vi "step loop.vi"(8 "error in (no error)":errorcluster, 11 "TapeDrive in":refnum<class "TapeDrive.lvclass">) -> (0 "error out":errorcluster, 1 "Boolean":bool, 2 "trajectories":dbl[][](graph)=[[1.0, 0.7046880791959296, 0.4965852858533471, 0.3499377259476329, 0.2465969370957652, 0.1737739140097176, 0.12245639698366893, 0.08629355394147512, 0.06081002915927391, 0.0628100291592739, 0.0648100291592739, 0.0668100291592739, 0.06881002915927391, 0.08881002915927391, 0.12881002915927392, 0.18881002915927392, 0.26881002915927393, 0.36881002915927397, 0.48881002915927396, 0.628810029159274, 0.788810029159274, 0.968810029159274, 1.0], [0.0, 0.0, 0.0, 0.0, 0.0, 0.0, 0.004000000000814907, 0.002999999998792191, 0.040000000000873115, 0.20499999999992724, 0.363999999999578, 0.5879999999997381, 0.7160000000003492, 0.7360000000007858, 0.7879999999986467, 0.6760000000012951, 0.3989999999994325, 0.01300000000082946, 0.004000000000814907, 0.003999999998995918, 0.0, 0.0, 0.0], [0.0, 0.0, 0.0, 0.0, 0.0, 0.0, 0.004000000000814907, -0.0010000000020227162, 0.037000000002080924, 0.16499999999905413, 0.15899999999965075, 0.22400000000016007, 0.12800000000061118, 0.020000000000436557, 0.05199999999786087, -0.11199999999735155, -0.27700000000186265, -0.385999999998603, -0.009000000000014552, -1.8189894035458565e-12, -0.003999999998995918, 0.0, 0.0]], 3 "TapeDrive out":refnum<class "TapeDrive.lvclass">, 4 "Slave":i32, 5 "VISA Refnum out":refnum<visa-resource-name>)   [LabVIEW 2020, in "TapeDrive.lvclass"]
uses:
  TapeDrive.lvclass
  TapeDrive.lvclass/TapeDrive.ctl
  shared/CompressAndUpdate(Poly)/CompressAndUpdate(Numeric).vi
  Newport ESP301/Newport ESP301.lvlib
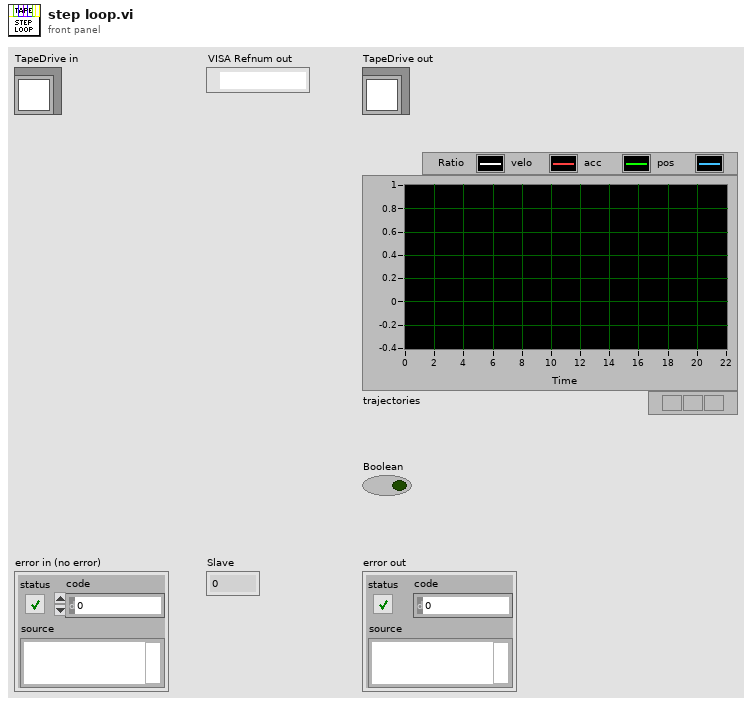
[diagram p1: front panel]
types:
  T1 = typedef "Direction_TypDef.ctl" = enum16{"left", "right"}
  T2 = cluster{"increase":dbl, "min velocity":dbl, "max velocity":dbl, "Stop increase":dbl}
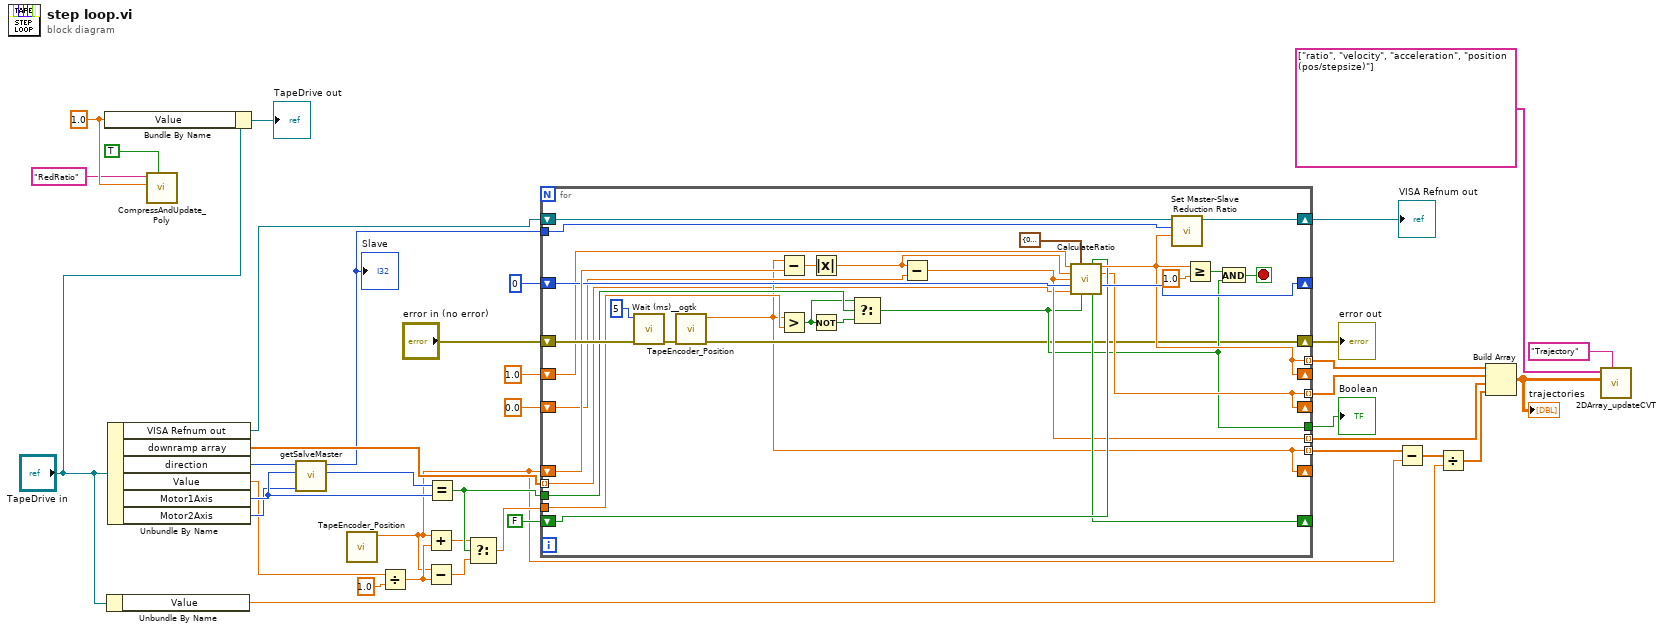
[diagram p0: block diagram]
diagram:
  w33 = 1.0 ("Reduction Ratio (0)")
  n1 = Bundle By Name(cluster="TapeDrive in", "Value"=w33) -> (→"TapeDrive out":refnum<class "TapeDrive.lvclass">)
  n2 = Unbundle By Name("TapeDrive in") -> ("Value"=w37:dbl)
  n3 = Unbundle By Name("TapeDrive in") -> ("VISA Refnum out"=w36:refnum<visa-resource-name>, "downramp array"=w35:dbl[], "direction"=w15:T1, "Value"=w18:dbl, "Motor1Axis"=w32:i32, "Motor2Axis"=w31:i32)
  n4 = call-poly "CompressAndUpdate_Poly.vi"("force CVT update (false)"=TRUE, "Numeric"=w33, "command or variable name"="RedRatio") -> ()  [unwired: 8 in, 1 out]
  n5 = call "getSalveMaster.vi"("Motor2Axis"=w31, "Motor1Axis"=w32, "direction"=w15) -> ("Master"=w29:i32, "Slave"=w27:i32)  [unwired: 7 in]
  "Slave" <- w27
  n6 = call "TapeEncoder_Position.vi"() -> ("position"=w1:dbl)  [unwired: 10 in, 1 out]
  n7 = Divide(x=w18, y=1.0) -> (x/y=w11:dbl)
  n8 = Add(x=w1, y=w11) -> (x+y=w3:dbl)
  n9 = Subtract(x=w1, y=w11) -> (x-y=w4:dbl)
  n10 = Equal?(x=w29, y=w32) -> (x = y?=w6:bool)
  n11 = Select(t=w3, s=w6, f=w4) -> (s? t:f=w5:dbl)
  n12 = for {
    shift-right: [w42] -> w28
    shift-left: "error in (no error)" -> [w66]
    tunnel: w27 -> [w67]
    shift-right: [w41] -> _
    shift-left: w1 -> [w64]
    shift-right: [w55] -> _
    shift-left: 1.0 -> [w54]
    tunnel: w5 -> [w62]
    tunnel: w6 -> [w60]
    shift-right: [w56] -> _
    shift-left: 0 -> [w57]
    tunnel: [w55] -> w8 mode=indexing
    tunnel: [w47] -> w9 mode=indexing
    tunnel: w35 -> [w39] mode=indexing
    shift-right: [w50] -> _
    shift-left: FALSE -> [w51]
    shift-right: [w47] -> _
    shift-left: 0.0 -> [w48]
    tunnel: [w46] -> w14 mode=indexing
    tunnel: [w41] -> w16 mode=indexing
    tunnel: [w44] -> w25
    shift-right: [w68] -> w26
    shift-left: w36 -> [w40]
    stop <- w52 stop-if-true
    n13 = call <userlib>:"Wait (ms)__ogtk.vi"("error in (no error)"=w66, "milliseconds to wait"=u32 5) -> ("error out"=w43:errorcluster)  [unwired: 8 in, 1 out]
    n14 = call "TapeEncoder_Position.vi"("error in (no error)"=w43) -> ("error IO"=w42:errorcluster, "position"=w41:dbl)  [unwired: 9 in]
    n15 = Subtract(x=w41, y=w64) -> (x-y=w63:dbl)
    n16 = Greater?(x=w41, y=w62) -> (0:w58:bool)
    n17 = Absolute Value(x=w63) -> (abs(x)=w49:dbl)
    n18 = Not(x=w58) -> (.not. x?=w59:bool)
    n19 = Select(t=w58, s=w60, f=w59) -> (s? t:f=w44:bool)
    n20 = Subtract(x=w49, y=w48) -> (x-y=w46:dbl)
    n21 = call "CalculateRatio.vi"("ratio"=w54, "Cluster"=T2 {"increase"=0.004, "min velocity"=0.1, "max velocity"=3.0, "Stop increase"=0.060000000000000005}, "decrease again"=w51, "velocity"=w49, "acceleration"=w46, "rep"=w57, "downramp"=w39, "stop"=w44) -> ("ratio out"=w55:dbl, "velocity out"=w47:dbl, "rep out"=w56:i32, "decrease again out"=w50:bool)  [unwired: 4 in]
    n22 = call "Set Master-Slave Reduction Ratio.vi"("Reduction Ratio (0)"=w55, "Axis (1)"=w67, "VISA resource name"=w40) -> ("VISA resource name out"=w68:refnum<visa-resource-name>)  [unwired: 3 in, 1 out]
    n23 = Greater Or Equal?(x=w55, y=1.0) -> (x >= y?=w53:bool)
    n24 = And(x=w53, y=w44) -> (x .and. y?=w52:bool)
  }
  "error out" <- w28
  "VISA Refnum out" <- w26
  "Boolean" <- w25
  n25 = Subtract(x=w16, y=w1) -> (x-y=w17:dbl[])
  n26 = Divide(x=w17, y=w37) -> (x/y=w19:dbl[])
  n27 = Build Array(w8, w9, w14, w19) -> (w21:dbl[][])
  "trajectories" <- w21
  n28 = call "2DArray_updateCVT.vi"("CVt_clusterName"="Trajectory", "trajectories"=w21, "Names"=string[] ["ratio", "velocity", "acceleration", "position (pos/stepsize)"]) -> ()  [unwired: 8 in, 1 out]
